vi "GetMeasures.vi"(8 "error in":errorcluster, 11 "StepRun in":refnum<class "StepRun.lvclass">) -> (0 "error out":errorcluster, 2 "Measures":refnum<class "Measure.lvclass">[](array[class]), 3 "StepRun out":refnum<class "StepRun.lvclass">)   [LabVIEW 2021, in "ProligentXMLGenerator.lvlib" / "StepRun.lvclass"]
doc: "Defines the value acquired by the measure."
uses:
  StepRun.lvclass
  StepRun.lvclass/StepRun.ctl
  Measure/Measure/Measure.lvclass
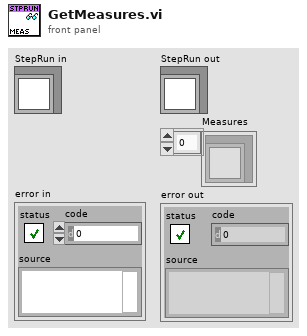
[diagram p1: front panel]
types:
  T1 = typedef "ProligentXMLGenerator.lvlib/StepRun.lvclass/Data.ctl" = cluster{"Name":string, "Measures":refnum<class "Measure.lvclass">[], "FailureReferences":refnum<class "FailureReference.lvclass">[], "Characteristics":refnum<class "Characteristic.lvclass">[], "Documents":refnum<class "Document.lvclass">[], "CustomData":refnum<class "CustomData.lvclass">, "StepExecutionStatus":refnum<class "ExecutionStatus.lvclass">, "StepRunId":refnum<class "Guid.lvclass">, "StepName":refnum<class "NonEmptyString_255.lvclass">, "StartDate":refnum<class "DateTime.lvclass">, "EndDate":refnum<class "DateTime.lvclass">, "TimeZoneInfoId":string}
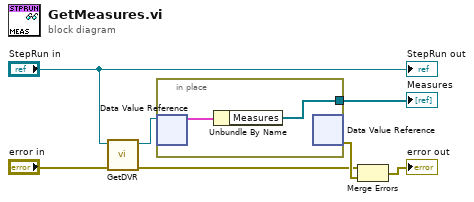
[diagram p0: block diagram]
diagram:
  n1 = call "GetDVR.vi"("error in"="error in", "StepRun"="StepRun in") -> ("error out"=w1:errorcluster, "DVRReference"=w6:refnum<data-value>)  [unwired: 8 in]
  n2 = in-place "In Place Element Structure" {
    in-place-border: [w8] -> w2
    n3 = in-place-dvr #1(w6) -> (w9:T1)  [unwired: 1 out]
    n4 = Unbundle By Name(w9) -> ("Measures"=w8:refnum<class "Measure.lvclass">[])
    n5 = in-place-dvr #1() -> (w7:errorcluster)  [unwired: 1 in, 1 out]
  }
  "Measures" <- w2
  n6 = Merge Errors(w1, w7) -> (→"error out":errorcluster)
  "StepRun out" <- "StepRun in"
